vi "PersonnelReportDataToGraph3d.vi"(8 "error in (no error)":errorcluster, 9 "Bar References":refnum<vi>[](array[refnum]), 10 "Pie References":refnum<vi>[](array[refnum]), 11 "Array":T1[](array[typedef])=[{"PersonnelName"="d1", "NumRequestsFulfilled"=11, "AvgFulfillTime(s)"=49.18181818181818, "NumReqWithAlarmFulfilled"=3, "NumRequestsAck"=9, "AvgAckTime(s)"=47.333333333333336, "NumReqWithAlarmAck"=2}, {"PersonnelName"="d2", "NumRequestsFulfilled"=1, "AvgFulfillTime(s)"=8.0, "NumReqWithAlarmFulfilled"=0, "NumRequestsAck"=1, "AvgAckTime(s)"=8.0, "NumReqWithAlarmAck"=0}, {"PersonnelName"="n1", "NumRequestsFulfilled"=3, "AvgFulfillTime(s)"=15.0, "NumReqWithAlarmFulfilled"=1, "NumRequestsAck"=2, "AvgAckTime(s)"=15.0, "NumReqWithAlarmAck"=1}, {"PersonnelName"="n2", "NumRequestsFulfilled"=5, "AvgFulfillTime(s)"=9.0, "NumReqWithAlarmFulfilled"=5, "NumRequestsAck"=3, "AvgAckTime(s)"=3.0, "NumReqWithAlarmAck"=0}]) -> (0 "error out":errorcluster, 1 "# Request with Alarm3":refnum<class "3D Plot Datatype.lvclass">[](array[class]), 2 "3Avg Time":refnum<class "3D Plot Datatype.lvclass">[](array[class]), 3 "Request Completed":refnum<class "3D Plot Datatype.lvclass">[](array[class]), 4 "Avg ACK Time":refnum<class "3D Plot Datatype.lvclass">[](array[class]), 5 "Pie Request Completed":refnum<class "3D Plot Datatype.lvclass">[](array[class]), 6 "Request Ack":refnum<class "3D Plot Datatype.lvclass">[](array[class]), 7 "Pie Request with Alarms":refnum<class "3D Plot Datatype.lvclass">[](array[class]))   [LabVIEW 2015]
uses:
  TypeDef/PersonnelReport.ctl
  <vilib>/Math Plots/3D Math Plots/3D Bar/3D Bar XCtrl/3D Bar.xctl
  <vilib>/Math Plots/3D Math Plots/3D Plot/3D Plot Datatype/3D Plot Datatype.lvclass
  <vilib>/Math Plots/3D Math Plots/3D Pie/3D Pie XCtrl/3D Pie.xctl
  <vilib>/Math Plots/3D Math Plots/3D Bar/3D Bar Datatype/Public/Plot Helper (Matrix).vi
  <vilib>/Math Plots/3D Math Plots/3D Pie/3D Pie Datatype/Public/Plot Helper (Vector).vi
  <vilib>/Math Plots/3D Math Plots/3D Bar/3D Bar Datatype/3D Bar Datatype.lvclass
  <vilib>/Math Plots/3D Math Plots/3D Pie/3D Pie Datatype/3D Pie Datatype.lvclass
panel:
  out "Request With Alarm":refnum<class "3D Plot Datatype.lvclass">[](xcontrol)
  out "Request Completed":refnum<class "3D Plot Datatype.lvclass">[](xcontrol)
  out "Avg ACK Time":refnum<class "3D Plot Datatype.lvclass">[](xcontrol)
  out "Request Ack":refnum<class "3D Plot Datatype.lvclass">[](xcontrol)
  out "# Request with Alarm":refnum<class "3D Plot Datatype.lvclass">[](xcontrol)
  out "Avg Time":refnum<class "3D Plot Datatype.lvclass">[](xcontrol)
  out "Request Completed":refnum<class "3D Plot Datatype.lvclass">[](xcontrol)
  out "Color and Name":cluster{"Color":u32, "String":string}[](array[cluster])
  out "Update":bool
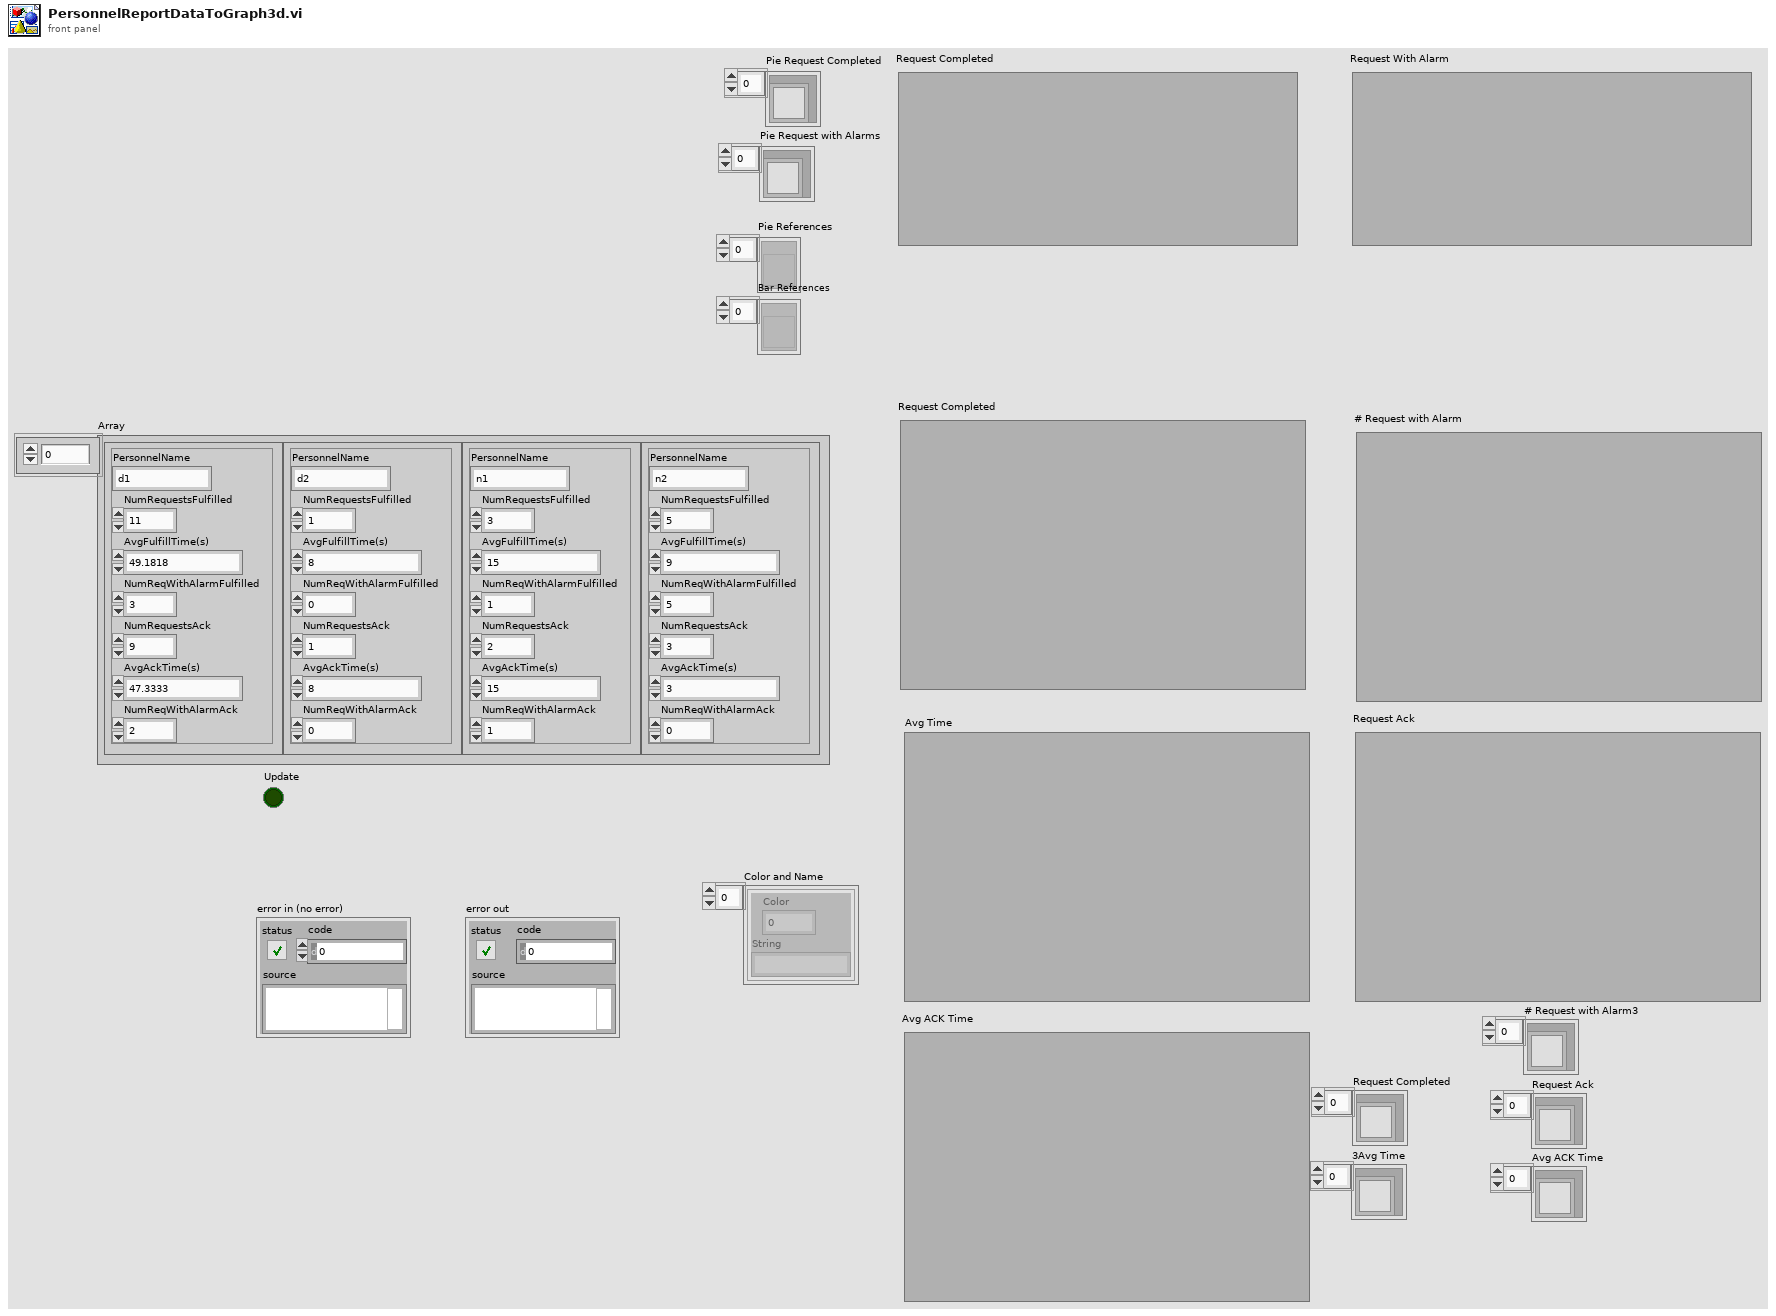
[diagram p1: front panel]
types:
  T1 = typedef "PersonnelReport.ctl" = cluster{"PersonnelName":string, "NumRequestsFulfilled":i32, "AvgFulfillTime(s)":dbl, "NumReqWithAlarmFulfilled":i32, "NumRequestsAck":i32, "AvgAckTime(s)":dbl, "NumReqWithAlarmAck":i32}
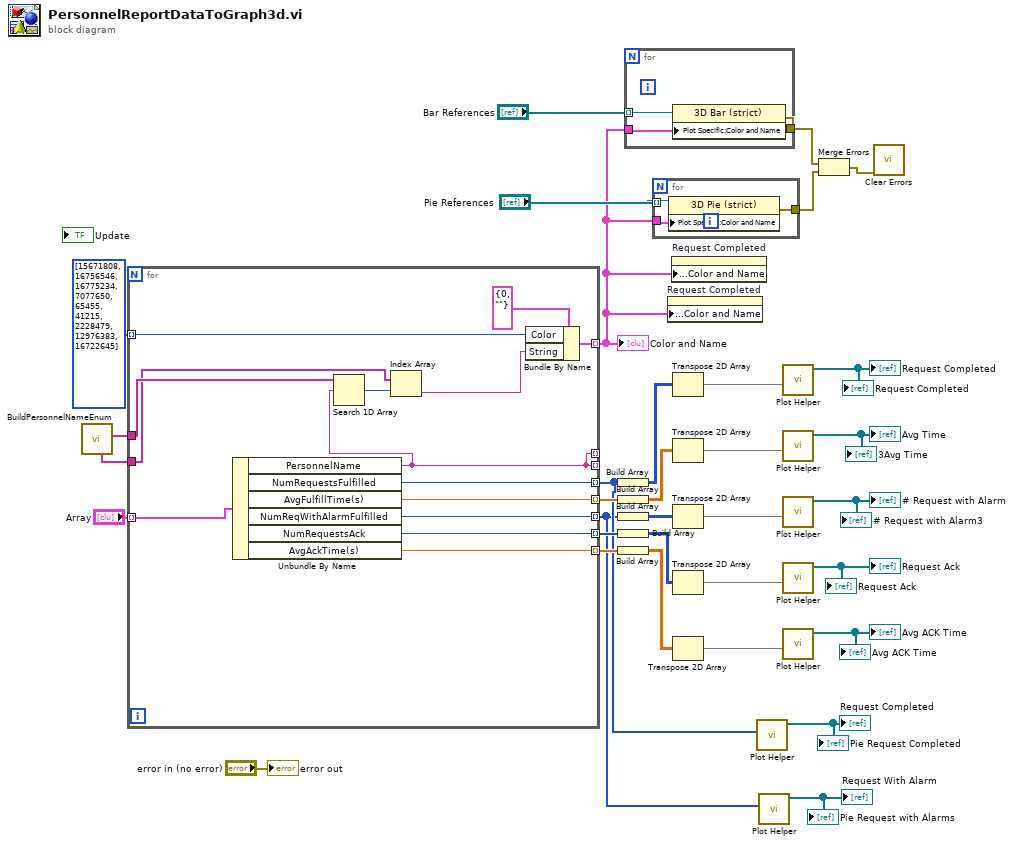
[diagram p0: block diagram]
diagram:
  n1 = call "BuildPersonnelNameEnum.vi"() -> ("PUIDs"=w2:string[], "Names"=w1:string[])  [unwired: 7 in, 3 out]
  n2 = for {
    tunnel: "Array" -> [w47] mode=indexing
    tunnel: [w35] -> _ mode=indexing
    tunnel: [w43] -> w11 mode=indexing
    tunnel: [w45] -> w6 mode=indexing
    tunnel: u32[] [15671808, 16756546, 16775234, 7077650, 65455, 41215, 2228479, 12976383, 16722645] -> [w44] mode=indexing
    tunnel: [w35] -> _ mode=indexing
    tunnel: [w42] -> w16 mode=indexing
    tunnel: [w41] -> w9 mode=indexing
    tunnel: [w40] -> w15 mode=indexing
    tunnel: [w39] -> w14 mode=indexing
    tunnel: w2 -> [w38]
    tunnel: w1 -> [w36]
    n3 = Unbundle By Name(w47) -> ("PersonnelName"=w35:string, "NumRequestsFulfilled"=w43:i32, "AvgFulfillTime(s)"=w42:dbl, "NumReqWithAlarmFulfilled"=w41:i32, "NumRequestsAck"=w40:i32, "AvgAckTime(s)"=w39:dbl)
    n4 = Search 1D Array(1D array=w38, element=w35) -> (index of element=w37:i32)  [unwired: 1 in]
    n5 = Index Array(array=w36, index=w37) -> (element=w34:string)
    n6 = Bundle By Name(cluster=cluster{"Color":u32, "String":string} {"Color"=0, "String"=""} ("Color Pair"), "Color"=w44, "String"=w34) -> (w45:cluster{"Color":u32, "String":string})
  }
  "Color and Name" <- w6
  n7 = Build Array(w11) -> (w30:i32[][])
  n8 = Build Array(w16) -> (w27:dbl[][])
  n9 = Build Array(w9) -> (w24:i32[][])
  n10 = Build Array(w15) -> (w21:i32[][])
  n11 = Build Array(w14) -> (w18:dbl[][])
  n12 = for {
    tunnel: "Bar References" -> [w50] mode=indexing
    tunnel: w6 -> [w49]
    tunnel: [w48] -> w5
    n13 = property class="3D Bar (strict)"(reference=w50, "Plot Specific:Color and Name"=w49) -> (error out=w48:errorcluster)  [unwired: 1 in, 1 out]
  }
  n14 = for {
    tunnel: "Pie References" -> [w53] mode=indexing
    tunnel: w6 -> [w52]
    tunnel: [w51] -> w4
    n15 = property class="3D Pie (strict)"(reference=w53, "Plot Specific:Color and Name"=w52) -> (error out=w51:errorcluster)  [unwired: 1 in, 1 out]
  }
  n16 = property on="Request Completed" class="3D Bar (strict)"("Plot Specific:Color and Name"=w6) -> ()  [unwired: 2 in, 2 out]
  n17 = property on="Request Completed" class="3D Pie (strict)"("Plot Specific:Color and Name"=w6) -> ()  [unwired: 2 in, 2 out]
  n18 = Transpose 2D Array(2D array=w30) -> (transposed array=w13:i32[][])
  n19 = Transpose 2D Array(2D array=w27) -> (transposed array=w28:dbl[][])
  n20 = Transpose 2D Array(2D array=w24) -> (transposed array=w23:i32[][])
  n21 = Transpose 2D Array(2D array=w21) -> (transposed array=w22:i32[][])
  n22 = Transpose 2D Array(2D array=w18) -> (transposed array=w17:dbl[][])
  n23 = call-poly <vilib>:"Plot Helper.vi"("x vector"=w11) -> ("3D Plot lvclass Array out"=→"Request Completed" →"Pie Request Completed":refnum<class "3D Plot Datatype.lvclass">[])  [unwired: 2 in, 8 out]
  n24 = call-poly <vilib>:"Plot Helper.vi"("x vector"=w9) -> ("3D Plot lvclass Array out"=→"Request With Alarm" →"Pie Request with Alarms":refnum<class "3D Plot Datatype.lvclass">[])  [unwired: 2 in, 8 out]
  n25 = call-poly <vilib>:"Plot Helper.vi"("z matrix"=w13) -> ("3D Plot lvclass Array out"=→"Request Completed" →"Request Completed":refnum<class "3D Plot Datatype.lvclass">[])  [unwired: 2 in, 8 out]
  n26 = call-poly <vilib>:"Plot Helper.vi"("z matrix"=w28) -> ("3D Plot lvclass Array out"=→"Avg Time" →"3Avg Time":refnum<class "3D Plot Datatype.lvclass">[])  [unwired: 2 in, 8 out]
  n27 = call-poly <vilib>:"Plot Helper.vi"("z matrix"=w23) -> ("3D Plot lvclass Array out"=→"# Request with Alarm" →"# Request with Alarm3":refnum<class "3D Plot Datatype.lvclass">[])  [unwired: 2 in, 8 out]
  n28 = call-poly <vilib>:"Plot Helper.vi"("z matrix"=w22) -> ("3D Plot lvclass Array out"=→"Request Ack" →"Request Ack":refnum<class "3D Plot Datatype.lvclass">[])  [unwired: 2 in, 8 out]
  n29 = call-poly <vilib>:"Plot Helper.vi"("z matrix"=w17) -> ("3D Plot lvclass Array out"=→"Avg ACK Time" →"Avg ACK Time":refnum<class "3D Plot Datatype.lvclass">[])  [unwired: 2 in, 8 out]
  n30 = Merge Errors(w5, w4) -> (w3:errorcluster)
  n31 = call <vilib>:"Clear Errors.vi"("error in (no error)"=w3) -> ()  [unwired: 5 in, 2 out]
  "error out" <- "error in (no error)"
